vi "Status_Var2String.vi"(10 "element":T1) -> (2 "resulting string":string)   [LabVIEW 2016]
uses:
  Status_VarsStruct.ctl
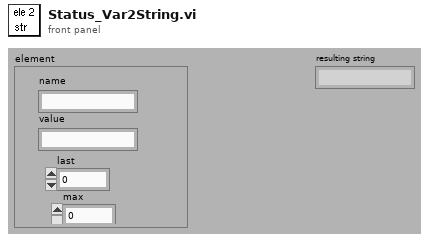
[diagram p1: front panel]
types:
  T1 = typedef "Status_VarsStruct.ctl" = cluster{"name":string, "value":string, "last":u32, "max":u32}
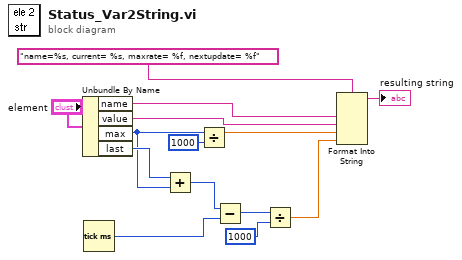
[diagram p0: block diagram]
diagram:
  n1 = Unbundle By Name("element") -> ("name"=w11:string, "value"=w10:string, "max"=w7:u32, "last"=w8:u32)
  n2 = Tick Count (ms)() -> (millisecond timer value=w5:u32)
  n3 = Add(x=w8, y=w7) -> (x+y=w6:u32)
  n4 = Divide(x=w7, y=u32 1000) -> (x/y=w9:dbl)
  n5 = Subtract(x=w6, y=w5) -> (x-y=w4:u32)
  n6 = Divide(x=w4, y=u32 1000) -> (x/y=w2:dbl)
  n7 = Format Into String(format string="name=%s, current= %s, maxrate= %f, nextupdate= %f", w11, w10, w9, w2) -> (resulting string=→"resulting string":string)  [unwired: 2 in, 1 out]
